vi "test4.vi"() -> ()   [LabVIEW 2023]
panel:
  out "error out":errorcluster
  out "return value":string
  in  "module path":path
  in  "error in (no error)":errorcluster
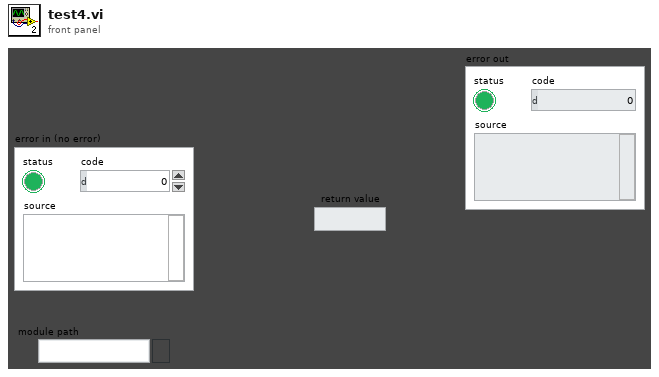
[diagram p1: front panel]
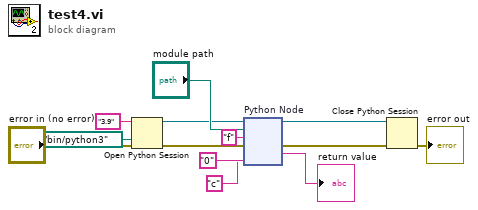
[diagram p0: block diagram]
diagram:
  n1 = Open Python Session(python version="3.9" ("Python version"), python path=path "/usr/bin/python3" ("Python path"), 3:"error in (no error)") -> (session out=w9:refnum<k35>, error out=w11:errorcluster)
  n2 = node "Python Node"(w9, "module path", "f" ("function name"), w11, "0", "c") -> (w8:refnum<k35>, w7:errorcluster, →"return value":string)  [unwired: 1 in, 2 out]
  n3 = Close Python Session(session in=w8, error in=w7) -> (11:→"error out":errorcluster)
